vi "Write Context.vi"(8 "error in":errorcluster, 10 "Context":refnum<class "State Pattern.lvclass">, 11 "State in":refnum<class "B State.lvclass">) -> (0 "error out":errorcluster, 3 "State out":refnum<class "B State.lvclass">)   [LabVIEW 2021, in "Context.lvlib" / "B State.lvclass"]
uses:
  B State.lvclass
  State Pattern/State Pattern/State Pattern.lvclass
  Context/Context.lvclass
  B State.lvclass/B State.ctl
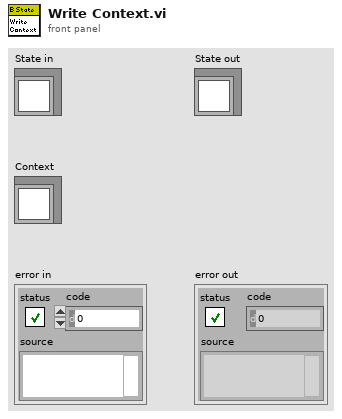
[diagram p1: front panel]
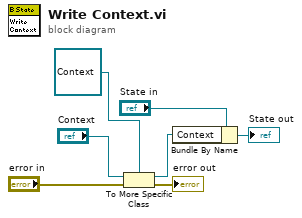
[diagram p0: block diagram]
diagram:
  n1 = To More Specific Class(target class=refnum<class "Context.lvclass"> refnum ("Context Actor.lvlib:Context Actor.lvclass"), reference="Context", error in="error in") -> (specific class reference=w7:refnum<class "Context.lvclass">, error out=→"error out":errorcluster)
  n2 = Bundle By Name(cluster="State in", "Context"=w7) -> (→"State out":refnum<class "B State.lvclass">)
